vi "ContextHelp_EnteringDialog.vi"(5 "error in (no error)":errorcluster) -> (15 "HelpStatus":bool, 19 "error out":errorcluster)   [LabVIEW 2012]
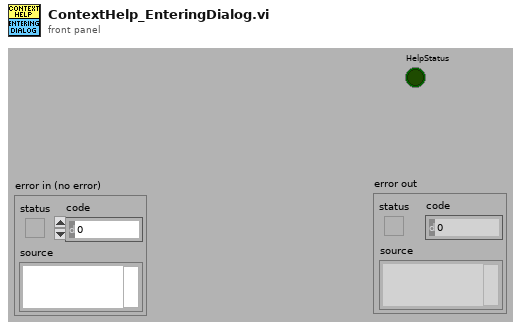
[diagram p1: front panel]
types:
  T1 = enum16{"SetPopUpEventTask", "GetStatus", "SetOpenState", "SetDialogCaller", "SetToolHelp"}
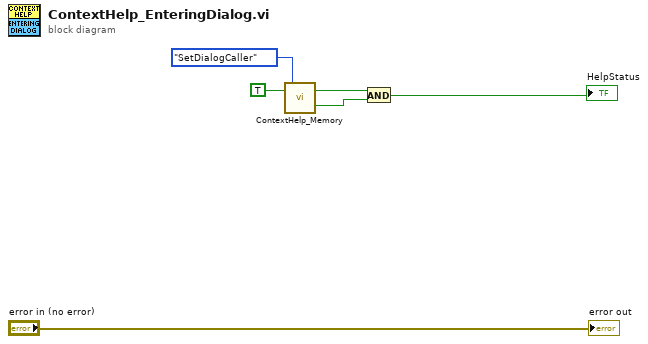
[diagram p0: block diagram]
diagram:
  n1 = call <resource>:"ContextHelp_Memory.vi"("State"=TRUE, "Actio(GetStatus)n"=T1."SetDialogCaller") -> ("Open"=w4:bool, "ToolHelp"=w3:bool)  [unwired: 2 in, 14 out]
  n2 = And(x=w4, y=w3) -> (x .and. y?=→"HelpStatus":bool)
  "error out" <- "error in (no error)"
